vi "Search and replace.vi"() -> ()   [LabVIEW 2015]
panel:
  in  "Skip lines":i32=1
  in  "Find-replace pairs":string[][](array[string])=[["\\s+", ","], [",,", ","], [",\\n", "\n"], ["^,", ""]]
  out "Output file":path
  in  "New file  extention":string="csv"
  out "Replaced text":string
  out "Original text":string
  in  "Input File":path
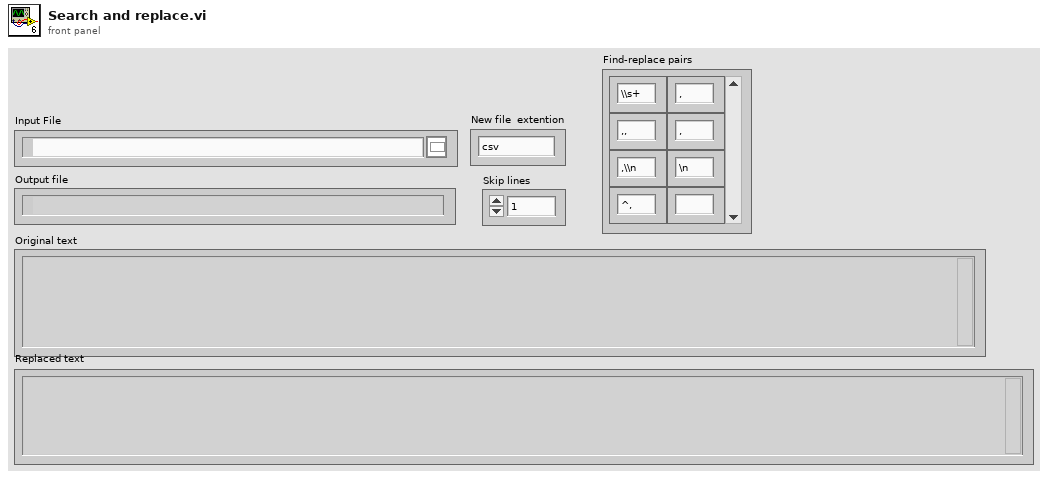
[diagram p1: front panel]
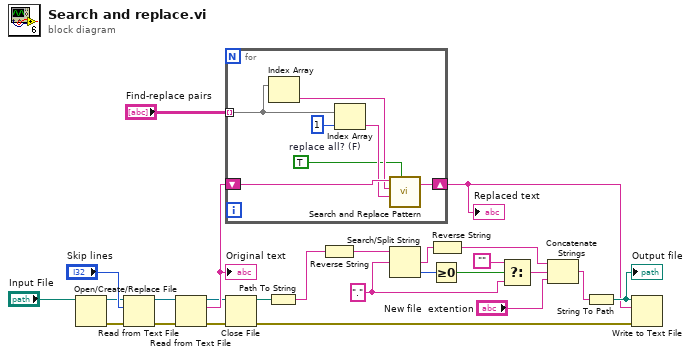
[diagram p0: block diagram]
diagram:
  w18 = "." ("search string/char (-)")
  n1 = Open/Create/Replace File(file path (use dialog)="Input File") -> (refnum out=w7:refnum<file>, error out=w9:errorcluster)  [unwired: 5 in, 1 out]
  n2 = Read from Text File(file (use dialog)=w7, count="Skip lines", error in=w9) -> (refnum out=w6:refnum<file>, error out=w5:errorcluster)  [unwired: 1 in, 2 out]
  n3 = Read from Text File(file (use dialog)=w6, error in=w5) -> (refnum out=w2:refnum<file>, text=w12:string, error out=w4:errorcluster)  [unwired: 2 in, 1 out]
  "Original text" <- w12
  n4 = for {
    tunnel: "Find-replace pairs" -> [w32] mode=indexing
    shift-right: [w26] -> w11
    shift-left: w12 -> [w30]
    w27 = TRUE  # replace all? (F)
    n5 = Index Array(array=w32) -> (element=w29:string)  [unwired: 1 in]
    n6 = Index Array(array=w32, index=1) -> (element=w28:string)
    n7 = call <vilib>:"Search and Replace Pattern.vi"("string"=w30, "regular expression (\"\")"=w29, "replace string (\"\")"=w28, "replace all? (F)"=w27) -> ("result string"=w26:string)  [unwired: 1 in, 1 out]
  }
  "Replaced text" <- w11
  n8 = Close File(refnum=w2, error in=w4) -> (path=w1:path, error out=w3:errorcluster)
  n9 = Path To String(path=w1) -> (string=w25:string)
  n10 = Reverse String(1:w25) -> (0:w24:string)
  n11 = Search/Split String(string=w24, search string/char (-)=w18) -> (match + rest of string=w22:string, offset of match=w23:i32)  [unwired: 1 in, 1 out]
  n12 = Greater Or Equal To 0?(x=w23) -> (x >= 0?=w20:bool)
  n13 = Reverse String(1:w22) -> (0:w21:string)
  n14 = Select(t="", s=w20, f=w18) -> (s? t:f=w17:string)
  n15 = Concatenate Strings(w21, w17, "New file  extention") -> (w15:string)
  n16 = String To Path(string=w15) -> (path=w14:path)
  "Output file" <- w14
  n17 = Write to Text File(file (use dialog)=w14, text=w11, error in=w3) -> ()  [unwired: 1 in, 3 out]
